vi "Request UI Display.vi"(6 "wait for reply (T)":bool=TRUE, 8 "error in (no error)":errorcluster, 10 "Scenario":T1, 11 "Module ID":i32=-1) -> (0 "error out":errorcluster, 3 "Accept?":bool)   [LabVIEW 2020, in "ExampleClone.lvlib"]
doc: "Requests another module to display its UI in the given <b>Display Scenario</b>: The \"Stand-Alone\" scenario asks the module to open its front panel as a new windows. The \"Managed\" scenario asks the module to broadcast a request for display which the UI Manager then processes, showing the module in its subpanel.\n____\nHAMPEL SOFTWARE ENGINEERING v2.6.0 (2023-12-19 10:54)"
uses:
  ExampleClone.lvlib
  Libraries/hse-libraries/Source/hse-dqmh/Controls/Module Display Scenarios.ctl
  Request UI Display Argument--cluster.ctl
  Request UI Display (Reply Payload)--cluster.ctl
  Libraries/hse-libraries/Source/hse-dqmh/hse-dqmh.lvlib
panel:
  out "timed out?":bool
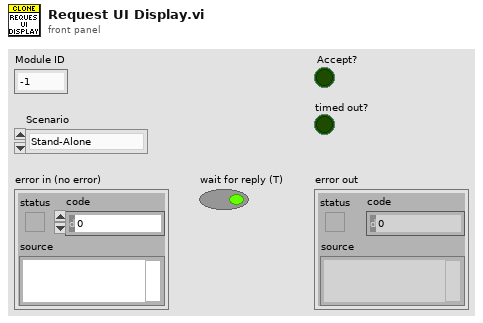
[diagram p1: front panel]
types:
  T1 = typedef "hse-dqmh.lvlib/Module Display Scenarios.ctl" = enum16{"Stand-Alone", "Managed"}
  T2 = typedef "ExampleClone.lvlib/Request UI Display Argument--cluster.ctl" = cluster{"Module ID":i32, "Scenario":T1, "Wait Notifier":refnum<notifier>, "wait for reply":bool}
  T3 = typedef "ExampleClone.lvlib/Request Events--cluster.ctl" = cluster{"Stop Module":refnum<user-event>, "Show Panel":refnum<user-event>, "Hide Panel":refnum<user-event>, "Show Diagram":refnum<user-event>, "Get Module Execution Status":refnum<user-event>, "Request UI Display":refnum<user-event>, "Configure":refnum<user-event>, "Prepare":refnum<user-event>, "ExampleMessage":refnum<user-event>}
  T4 = typedef "ExampleClone.lvlib/Request UI Display (Reply Payload)--cluster.ctl" = cluster{"Accept?":bool, "error":errorcluster, "Module ID":i32}
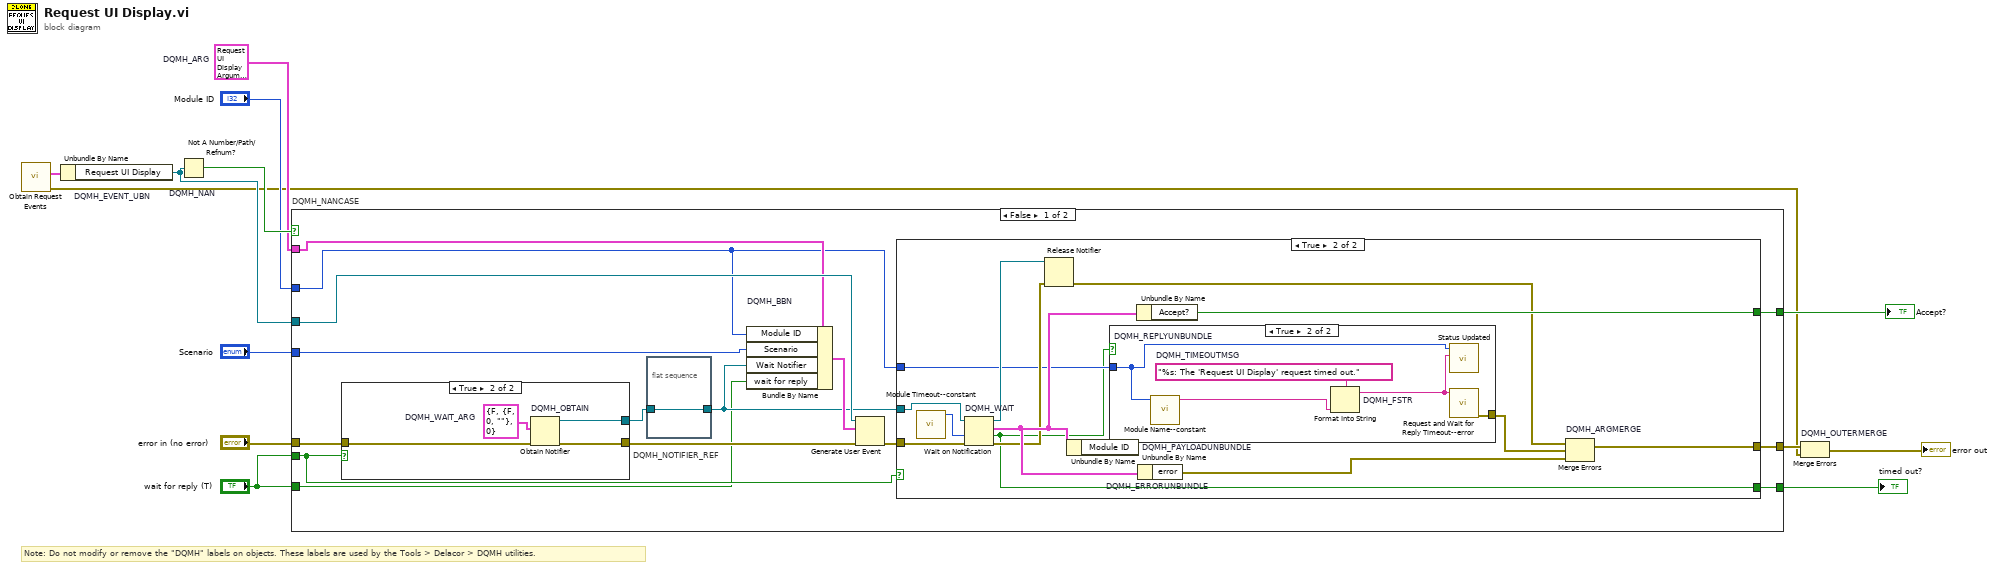
[diagram p0: block diagram]
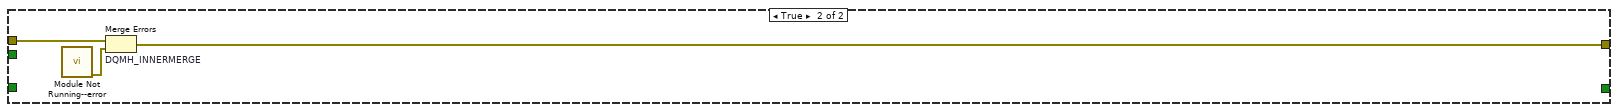
[diagram p5: hidden frame]
diagram:
  w7 = T2 {"Module ID"=-1, "Scenario"=enum."Stand-Alone", "Wait Notifier"=refnum, "wait for reply"=FALSE}  # DQMH_ARG
  # "Note: Do not modify or remove the \"DQMH\" labels on objects. These labels are used by the Tools > Delacor > DQMH utilities."
  n1 = call "Obtain Request Events.vi"() -> ("error out"=w3:errorcluster, "ExampleClone Request Events"=w2:T3)  [unwired: 10 in]
  n2 = Unbundle By Name "DQMH_EVENT_UBN"(w2) -> ("Request UI Display"=w8:refnum<user-event>)
  n3 = Not A Number/Path/Refnum? "DQMH_NAN"(number/path/refnum=w8) -> (NaN/Path/Refnum?=w9:bool)
  n4 = case "DQMH_NANCASE" shown="False" w9 {
    tunnel: "error in (no error)" -> [w28 w56]
    tunnel: w8 -> [w26 _]
    tunnel: [w23 w55] -> w10
    tunnel: [w24 _] -> w12
    tunnel: "wait for reply (T)" -> [w21 _]
    tunnel: w7 -> [w18 _]
    tunnel: "Module ID" -> [w15 _]
    tunnel: "Scenario" -> [w17 _]
    tunnel: "wait for reply (T)" -> [w16 _]
    tunnel: [w14 _] -> w1
    frame False {
      n5 = case shown="True" w21 {
        tunnel: w28 -> [w49 w53]
        tunnel: [w49 w52] -> w25
        tunnel: [_ w50] -> w20
        frame False {
        }
        frame True {
          w51 = T4 {"Accept?"=FALSE, "error"={"status"=FALSE, "code"=0, "source"=""}, "Module ID"=0}  # DQMH_WAIT_ARG
          n6 = Obtain Notifier "DQMH_OBTAIN"(notification data type=w51, error in (no error)=w53) -> (notifier out=w50:refnum<notifier>, error out=w52:errorcluster)  [unwired: 2 in, 1 out]
        }
      }
      n7 = flat-sequence "DQMH_NOTIFIER_REF" {
        tunnel: w20 -> [w29]
        tunnel: [w29] -> w19
        frame #0 {
        }
      }
      n8 = Bundle By Name "DQMH_BBN"(cluster=w18, "Module ID"=w15, "Scenario"=w17, "Wait Notifier"=w19, "wait for reply"=w16) -> (w22:T2)
      n9 = Generate User Event(user event=w26, event data cluster=w22, error in=w25) -> (error out=w27:errorcluster)  [unwired: 1 in, 1 out]
      n10 = case shown="True" w21 {
        tunnel: w27 -> [w30 w43]
        tunnel: w19 -> [_ w42]
        tunnel: [_ w36] -> w24
        tunnel: [w30 w40] -> w23
        tunnel: w15 -> [_ w32]
        tunnel: [_ w31] -> w14
        frame False {
        }
        frame True {
          n11 = call "Module Timeout--constant.vi"() -> ("Module Timeout"=w38:i32)  [unwired: 11 in]
          n12 = Wait on Notification "DQMH_WAIT"(notifier=w42, timeout in ms (-1)=w38, error in (no error)=w43) -> (notifier out=w41:refnum<notifier>, notification=w37:T4, timed out?=w31:bool, error out=w35:errorcluster)  [unwired: 1 in]
          n13 = Release Notifier(notifier=w41, error in (no error)=w35) -> (error out=w34:errorcluster)  [unwired: 1 in, 2 out]
          n14 = Unbundle By Name "DQMH_PAYLOADUNBUNDLE"(w37) -> ()  [unwired: 1 out]
          n15 = case shown="True" w31 {
            tunnel: [_ w46] -> w33
            tunnel: w32 -> [_ w44]
            frame False {
            }
            frame True {
              w48 = "%s: The 'Request UI Display' request timed out."  # DQMH_TIMEOUTMSG
              n16 = call "Module Name--constant.vi"("Module ID"=w44) -> ("Module Name"=w45:string)  [unwired: 10 in]
              n17 = Format Into String "DQMH_FSTR"(format string=w48, w45) -> (resulting string=w47:string)  [unwired: 2 in, 1 out]
              n18 = call "Status Updated.vi"("Status"=w47, "Module ID"=w44) -> ()  [unwired: 9 in, 1 out]
              n19 = call "Request and Wait for Reply Timeout--error.vi"("Error Message"=w47) -> ("error out"=w46:errorcluster)  [unwired: 10 in]
            }
          }
          n20 = Unbundle By Name "DQMH_REPLYUNBUNDLE"(w37) -> ("Accept?"=w36:bool)
          n21 = Unbundle By Name "DQMH_ERRORUNBUNDLE"(w37) -> ("error"=w39:errorcluster)
          n22 = Merge Errors "DQMH_ARGMERGE"(w34, w33, w39) -> (w40:errorcluster)
        }
      }
    }
    frame True {
      n23 = call "Module Not Running--error.vi"() -> ("error out"=w54:errorcluster)  [unwired: 11 in]
      n24 = Merge Errors "DQMH_INNERMERGE"(w56, w54) -> (w55:errorcluster)
    }
  }
  "Accept?" <- w12
  "timed out?" <- w1
  n25 = Merge Errors "DQMH_OUTERMERGE"(w10, w3) -> (→"error out":errorcluster)
